vi "Define Events.vi"(8 "error in (no error)":errorcluster, 11 "Controller Actor in":refnum<class "Controller Actor.lvclass">) -> (0 "error out":errorcluster, 3 "Controller Actor out":refnum<class "Controller Actor.lvclass">)   [LabVIEW 2017, in "Event Actors.lvlib" / "Controller Actor.lvclass"]
doc: "This dynamic dispatch VI has to be overriden by the concrete Controller Actor subclasses in order to define the event served by the Controller."
uses:
  Controller Actor.lvclass
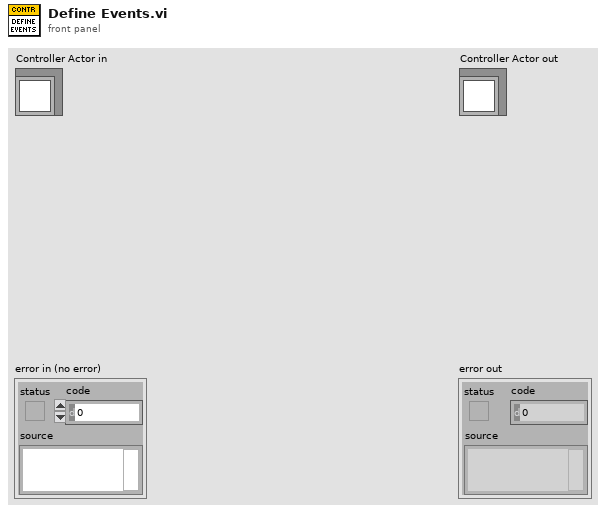
[diagram p1: front panel]
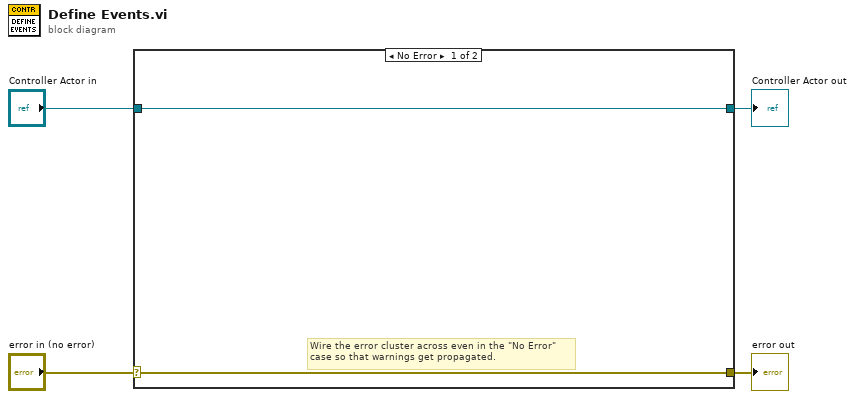
[diagram p0: block diagram]
diagram:
  n1 = case shown="No Error" "error in (no error)" {
    selector: "error in (no error)" -> [w5 w8]
    tunnel: [w5 w8] -> w3
    tunnel: [w6 w7] -> w1
    tunnel: "Controller Actor in" -> [w6 w7]
    frame No Error {
      # "Wire the error cluster across even in the \"No Error\"\ncase so that warnings get propagated."
    }
    frame Error {
    }
  }
  "error out" <- w3
  "Controller Actor out" <- w1
